vi "CreateLimitsRegisters.vi"() -> (4 "LimitsRegisters":T1={"HighLimits"="HighLimits", "LowLimits"="LowLimits", "ClearLimits"="ClearLimits", "LimitsFlag"="ClearLimits"})   [LabVIEW 2017, in "ScaleAndLimit.lvlib"]
doc: "Creates limit registers."
uses:
  ScaleAndLimit.lvlib
  LimitsRegisters.ctl
  <vilib>/rvi/eio/common/nirviEmuReportErrorAndStop.vi
  <vilib>/rvi/DataTransferAndStorage/Container/Common/niFpgaContainerSetEmuInfo.vi
  <vilib>/rvi/DataTransferAndStorage/Container/Common/niFpgaContainerGetUniqueNameForEmu.vi
  <vilib>/rvi/LocalResourceManager/LocalResourceManager.xnode
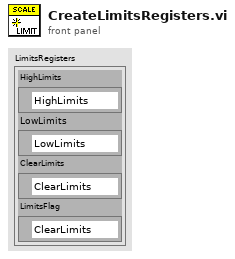
[diagram p1: front panel]
types:
  T1 = typedef "ScaleAndLimit.lvlib/LimitsRegisters.ctl" = cluster{"HighLimits":refnum<k21>, "LowLimits":refnum<k21>, "ClearLimits":refnum<k21>, "LimitsFlag":refnum<k21>}
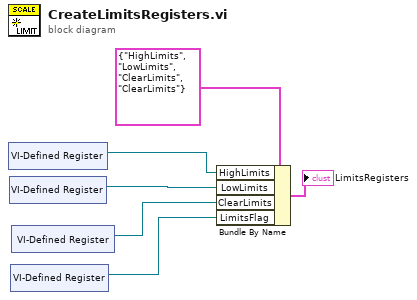
[diagram p0: block diagram]
diagram:
  n1 = xnode "VI-Defined Register"() -> ("Register Out"=w5:refnum<k21>)
  n2 = xnode "VI-Defined Register"() -> ("Register Out"=w4:refnum<k21>)
  n3 = xnode "VI-Defined Register"() -> ("Register Out"=w1:refnum<k21>)
  n4 = xnode "VI-Defined Register"() -> ("Register Out"=w2:refnum<k21>)
  n5 = Bundle By Name(cluster=T1 {"HighLimits"="HighLimits", "LowLimits"="LowLimits", "ClearLimits"="ClearLimits", "LimitsFlag"="ClearLimits"} ("LimitsRegisters"), "HighLimits"=w5, "LowLimits"=w4, "ClearLimits"=w2, "LimitsFlag"=w1) -> (→"LimitsRegisters":T1)
